vi "TWM Client Cmd Get Algorithm Info.vi"(7 "end of packet key":string="TWM:command:EndOfPacket", 8 "error in":errorcluster, 10 "algorithm id":string, 11 "handle":i32) -> (0 "error out":errorcluster, 2 "algorithm info":T1, 3 "handle out":i32)   [LabVIEW 2020, in "TWM Client.lvlib"]
doc: "Write Get algorithm info command packet to TWM server. Get answer."
uses:
  TWM Client.lvlib
  TWM Client Algorithm Info.ctl
  octave/infolib/String.vi
  octave/infolib/Get 1D String.vi
  <vilib>/Utility/error.llb/Error Cluster From Error Code.vi
  octave/infolib/GetBoolean.vi
  octave/infolib/GetString.vi
  <vilib>/ErrorRing/Error Ring.xnode
  octave/infolib/infolib.lvlib
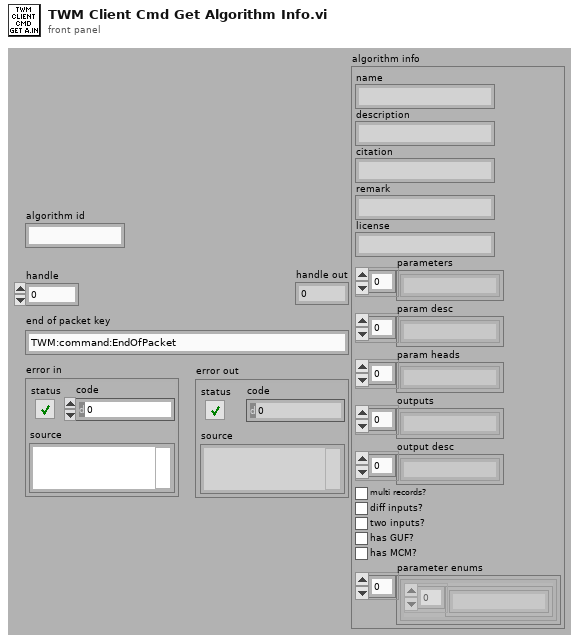
[diagram p1: front panel]
types:
  T1 = typedef "TWM Client.lvlib/TWM Client Algorithm Info.ctl" = cluster{"name":string, "description":string, "citation":string, "remark":string, "license":string, "parameters":string[], "param desc":string[], "param heads":string[], "outputs":string[], "output desc":string[], "multi records?":bool, "diff inputs?":bool, "two inputs?":bool, "has GUF?":bool, "has MCM?":bool, "parameter enums":cluster{"parameter enums":string[]}[]}
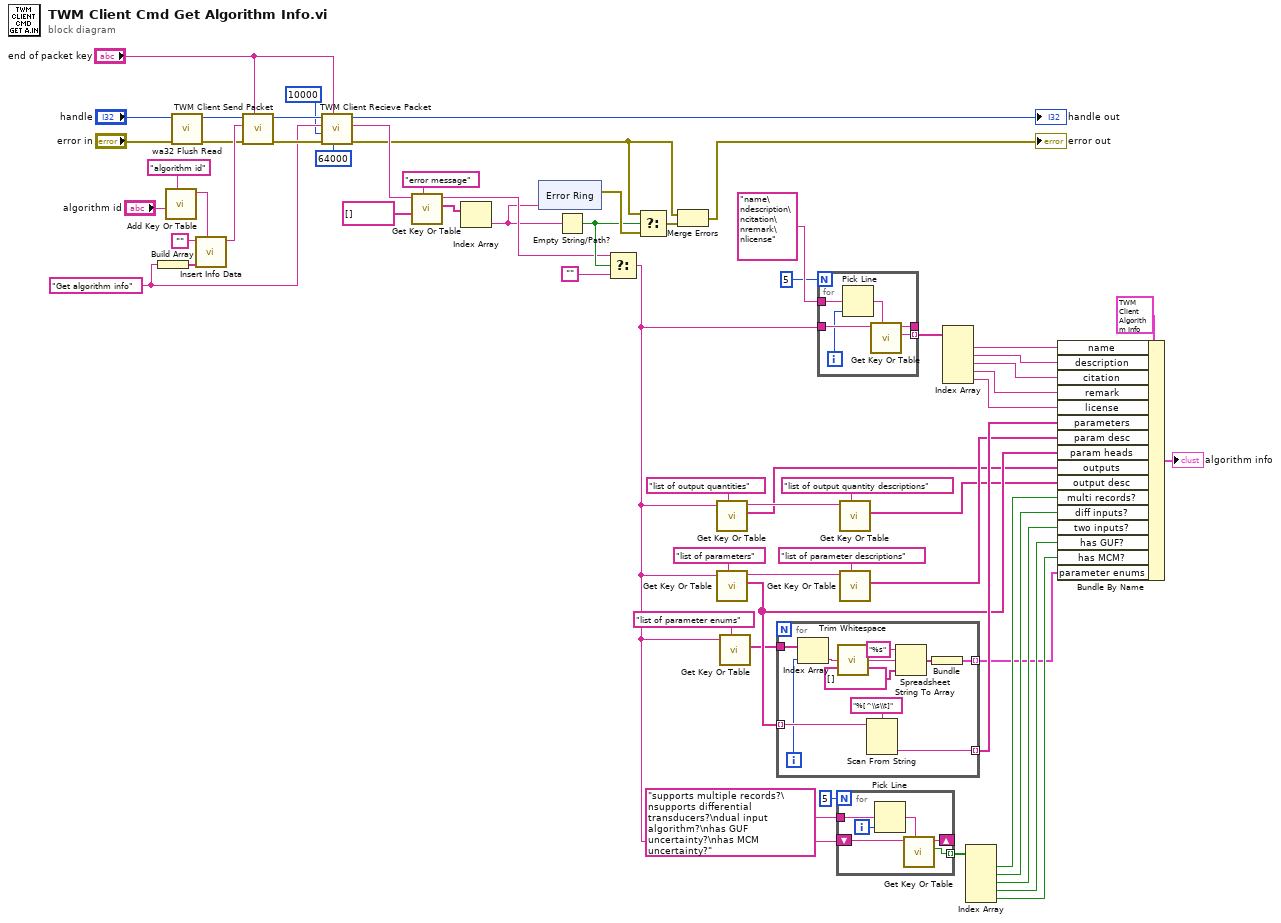
[diagram p0: block diagram]
diagram:
  w52 = "Get algorithm info" ("key string")
  n1 = Build Array(w52) -> (w53:string[])
  n2 = call-poly "Add Key Or Table.vi"("key description"="algorithm id", "string"="algorithm id") -> ("info data out"=w54:string)  [unwired: 8 in, 1 out]
  n3 = call "wa32 Flush Read.vi"("error in"="error in", "handle"="handle") -> ("error out"=w7:errorcluster, "handle out"=w6:i32)  [unwired: 7 in, 1 out]
  n4 = call "Insert Info Data.vi"("info data to insert"=w54, "sections"=w53, "info data"="") -> ("info data out"=w51:string)  [unwired: 7 in, 1 out]
  n5 = call "TWM Client Send Packet.vi"("end of packet key"="end of packet key", "error in"=w7, "command string"=w51, "handle"=w6) -> ("error out"=w61:errorcluster, "handle out"=w59:i32)  [unwired: 6 in]
  n6 = call "TWM Client Recieve Packet.vi"("max message length (1024)"=64000, "end of packet key"="end of packet key", "error in"=w61, "timeout [ms] (5000 ms)"=10000, "message header (empty)"=w52, "handle in"=w59) -> ("error out"=w46:errorcluster, "message data"=w56:string, "handle out"=→"handle out":i32)  [unwired: 3 in]
  n7 = call-poly "Get Key Or Table.vi"("key description"="error message", "string"=string[] [], "info data"=w56) -> ("value"=w47:string[], "info data out"=w43:string)  [unwired: 5 in, 2 out]
  n8 = Index Array(array=w47) -> (element=w9:string)  [unwired: 1 in]
  n9 = xnode "Error Ring"("parameter 0"=w9) -> ("error out"=w45:errorcluster)
  n10 = Empty String/Path?(string/path=w9) -> (empty?=w44:bool)
  n11 = Select(t=w43, s=w44, f="") -> (s? t:f=w4:string)
  n12 = Select(t=w46, s=w44, f=w45) -> (s? t:f=w50:errorcluster)
  n13 = Merge Errors(w46, w50) -> (→"error out":errorcluster)
  n14 = call-poly "Get Key Or Table.vi"("key description"="list of output quantities", "info data"=w4) -> ("value"=w20:string[], "info data out"=w22:string)  [unwired: 6 in, 2 out]
  n15 = call-poly "Get Key Or Table.vi"("key description"="list of parameters", "info data"=w4) -> ("value"=w26:string[], "info data out"=w37:string)  [unwired: 6 in, 2 out]
  n16 = call-poly "Get Key Or Table.vi"("key description"="list of parameter enums", "info data"=w4) -> ("value"=w2:string[])  [unwired: 6 in, 3 out]
  n17 = for {
    tunnel: w26 -> [w73] mode=indexing
    tunnel: [w71] -> w28 mode=indexing
    tunnel: w2 -> [w70]
    tunnel: [w64] -> w1 mode=indexing
    i -> [w69]
    n18 = Index Array(array=w70, index=w69) -> (element=w68:string)
    n19 = call <vilib>:"Trim Whitespace.vi"("string"=w68) -> ("trimmed string"=w63:string)  [unwired: 1 in]
    n20 = Scan From String(format string="%[^\\s\\t]", input string=w73) -> (output 1=w71:string)  [unwired: 3 in, 3 out]
    n21 = Spreadsheet String To Array(format string="%s", spreadsheet string=w63, array type (2D Dbl)=string[] []) -> (array=w65:string[])  [unwired: 1 in]
    n22 = Bundle(w65) -> (w64:cluster{string[]})  [unwired: 1 in]
  }
  n23 = for {
    N: 5 -> [_]
    tunnel: [w79] -> _
    tunnel: w4 -> [w78]
    tunnel: [w77] -> w35 mode=indexing
    tunnel: "name\ndescription\ncitation\nremark\nlicense" -> [w76]
    i -> [w74]
    n24 = Pick Line(multi-line string=w76, line index=w74) -> (output string=w75:string)  [unwired: 1 in]
    n25 = call-poly "Get Key Or Table.vi"("key description"=w75, "info data"=w78) -> ("value"=w77:string, "info data out"=w79:string)  [unwired: 6 in, 2 out]
  }
  n26 = for {
    N: 5 -> [_]
    tunnel: "supports multiple records?\nsupports differential transducers?\ndual input algorithm?\nhas GUF uncertainty?\nhas MCM uncertainty?" -> [w83]
    shift-right: [w84] -> _
    shift-left: w4 -> [w85]
    tunnel: [w80] -> w17 mode=indexing
    i -> [w81]
    n27 = Pick Line(multi-line string=w83, line index=w81) -> (output string=w82:string)  [unwired: 1 in]
    n28 = call-poly "Get Key Or Table.vi"("key description"=w82, "info data"=w85) -> ("value"=w80:bool, "info data out"=w84:string)  [unwired: 6 in, 2 out]
  }
  n29 = call-poly "Get Key Or Table.vi"("key description"="list of output quantity descriptions", "info data"=w22) -> ("value"=w19:string[])  [unwired: 6 in, 3 out]
  n30 = call-poly "Get Key Or Table.vi"("key description"="list of parameter descriptions", "info data"=w37) -> ("value"=w27:string[])  [unwired: 6 in, 3 out]
  n31 = Index Array(array=w35) -> (element #1=w33:string, element #2=w32:string, element #3=w31:string, element #4=w30:string, element #5=w29:string)  [unwired: 5 in]
  n32 = Index Array(array=w17) -> (element #1=w16:bool, element #2=w15:bool, element #3=w14:bool, element #4=w12:bool, element #5=w11:bool)  [unwired: 5 in]
  n33 = Bundle By Name(cluster=T1 {"name"="", "description"="", "citation"="", "remark"="", "license"="", "parameters"=[], "param desc"=[], "param heads"=[], "outputs"=[], "output desc"=[], "multi records?"=FALSE, "diff inputs?"=FALSE, "two inputs?"=FALSE, "has GUF?"=FALSE, "has MCM?"=FALSE, "parameter enums"=[]} ("alg info"), "name"=w33, "description"=w32, "citation"=w31, "remark"=w30, "license"=w29, "parameters"=w28, "param desc"=w27, "param heads"=w26, "outputs"=w20, "output desc"=w19, "multi records?"=w16, "diff inputs?"=w15, "two inputs?"=w14, "has GUF?"=w12, "has MCM?"=w11, "parameter enums"=w1) -> (→"algorithm info":T1)
